vi "Read Base Actor Notifiers.vi"(11 "Template in":refnum<class "Template.lvclass">) -> (3 "Base Actor Notifiers":T1)   [LabVIEW 2020, in "Template.lvlib" / "Template.lvclass"]
uses:
  Template.lvclass
  typedefs/base actor notifiers.ctl
  Template.lvclass/Template.ctl
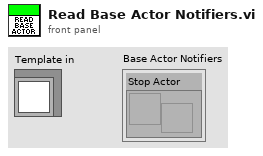
[diagram p1: front panel]
types:
  T1 = typedef "Template.lvlib/Template.lvclass/base actor notifiers.ctl" = cluster{"Stop Actor":refnum<notifier>}
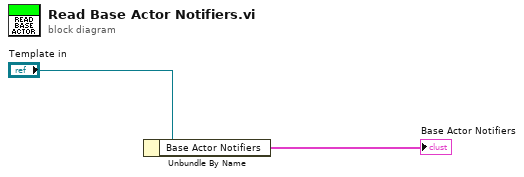
[diagram p0: block diagram]
diagram:
  n1 = Unbundle By Name("Template in") -> ("Base Actor Notifiers"=→"Base Actor Notifiers":T1)
